vi "Project.vi"() -> ()   [LabVIEW 2023]
uses:
  <vilib>/addons/Biomedical/Biosignal Measurements/EEG/subVIs/bmt_EEG Frequency-domain Measures.ctl
  <vilib>/addons/Biomedical/Biosignal Measurements/EEG/EEG FFT Spectrum (Waveform).vi
  <vilib>/addons/Biomedical/NI_BMTK_Measurements.lvlib
  <vilib>/Analysis/NI_AALBase.lvlib
panel:
  out "beta standard deviation":dbl format="%0.2f"
  out "beta mean":dbl format="%0.2f"
  out "alpha standard deviation":dbl format="%0.2f"
  out "alpha mean":dbl format="%0.2f"
  out "theta standard deviation":dbl format="%0.2f"
  out "theta mean":dbl format="%0.2f"
  out "delta standard deviation":dbl format="%0.2f"
  out "delta mean":dbl format="%0.2f"
  out "frequency measurements":T1
  out "FFT spectrum":cluster{"f0":dbl, "df":dbl, "S(f)":dbl[]}
  out "EEG in 10s":dbl[](graph)
  out "EEG in 1s":waveform(dbl)(graph)
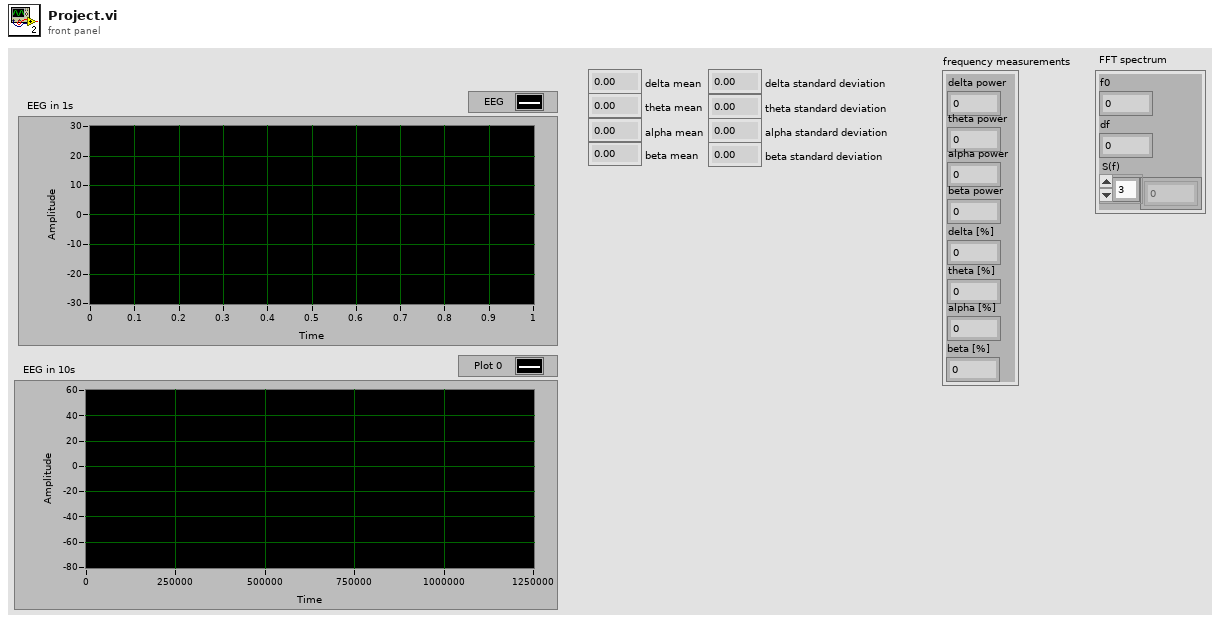
[diagram p1: front panel]
types:
  T1 = typedef "NI_BMTK_Measurements.lvlib/bmt_EEG Frequency-domain Measures.ctl" = cluster{"delta power":dbl, "theta power":dbl, "alpha power":dbl, "beta power":dbl, "delta [%]":dbl, "theta [%]":dbl, "alpha [%]":dbl, "beta [%]":dbl}
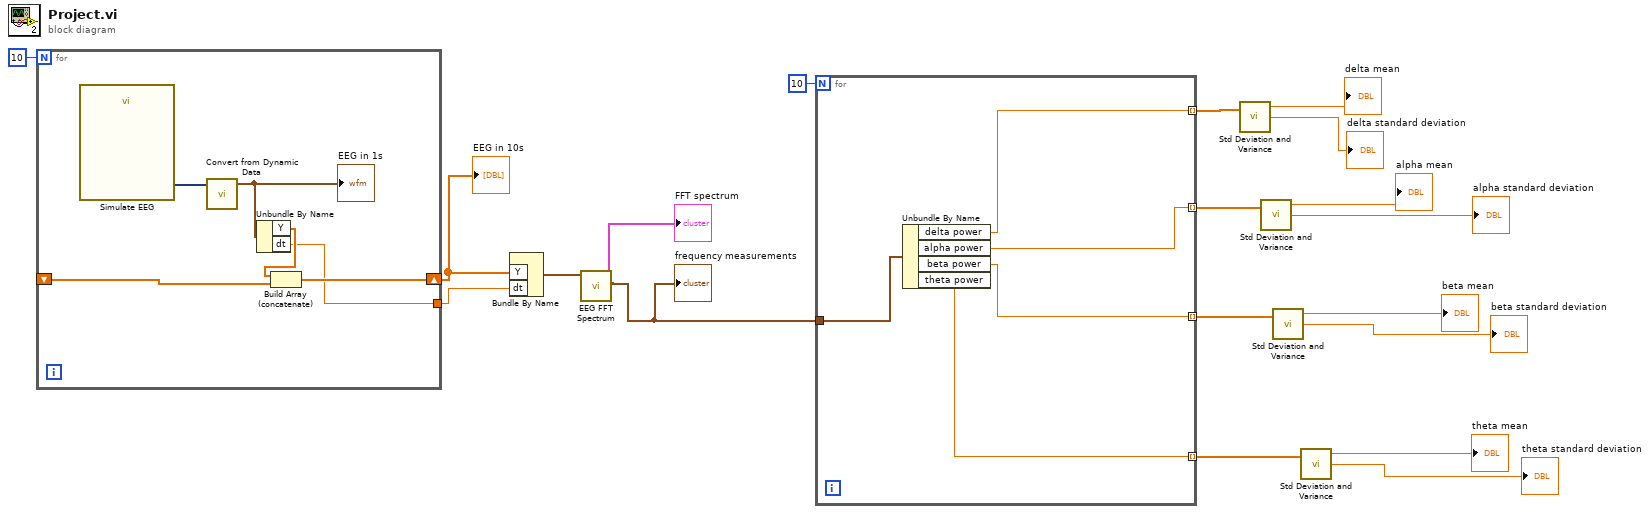
[diagram p0: block diagram]
diagram:
  n1 = for {
    N: 10 -> [_]
    shift-right: [w22] -> w18
    shift-left: _ -> [w21]
    tunnel: [w20] -> w17
    n2 = call "Simulate EEG"() -> ("EEG"=w25:dynamicdata)  [unwired: 10 in, 1 out]
    n3 = call "Convert from Dynamic Data"("Dynamic Data Type"=w25) -> ("Waveform"=w24:waveform(dbl))  [unwired: 3 in]
    "EEG in 1s" <- w24
    n4 = Unbundle By Name(w24) -> ("Y"=w23:dbl[], "dt"=w20:dbl)
    n5 = Build Array (concatenate)(w23, w21) -> (w22:dbl[])
  }
  "EEG in 10s" <- w18
  n6 = Bundle By Name("Y"=w18, "dt"=w17) -> (w5:waveform(dbl))  [unwired: 1 in]
  n7 = call-poly <vilib>:"EEG FFT Spectrum.vi"("EEG"=w5) -> ("frequency measurements"=w1:T1, "FFT spectrum"=→"FFT spectrum":cluster{"f0":dbl, "df":dbl, "S(f)":dbl[]})  [unwired: 8 in, 1 out]
  "frequency measurements" <- w1
  n8 = for {
    N: 10 -> [_]
    tunnel: w1 -> [w30]
    tunnel: [w29] -> w6 mode=indexing
    tunnel: [w28] -> w4 mode=indexing
    tunnel: [w27] -> w3 mode=indexing
    tunnel: [w26] -> w2 mode=indexing
    n9 = Unbundle By Name(w30) -> ("delta power"=w29:dbl, "alpha power"=w28:dbl, "beta power"=w27:dbl, "theta power"=w26:dbl)
  }
  n10 = call <vilib>:"Std Deviation and Variance.vi"("X"=w6) -> ("mean"=→"delta mean":dbl, "standard deviation"=→"delta standard deviation":dbl)  [unwired: 1 in, 1 out]
  n11 = call <vilib>:"Std Deviation and Variance.vi"("X"=w4) -> ("mean"=→"alpha mean":dbl, "standard deviation"=→"alpha standard deviation":dbl)  [unwired: 1 in, 1 out]
  n12 = call <vilib>:"Std Deviation and Variance.vi"("X"=w3) -> ("mean"=→"beta mean":dbl, "standard deviation"=→"beta standard deviation":dbl)  [unwired: 1 in, 1 out]
  n13 = call <vilib>:"Std Deviation and Variance.vi"("X"=w2) -> ("mean"=→"theta mean":dbl, "standard deviation"=→"theta standard deviation":dbl)  [unwired: 1 in, 1 out]
